vi "JSON File to Cluster.vi"(7 "Cluster (Data Type)":variant, 11 "JSON Document":path) -> (2 "Data":variant)   [LabVIEW 2013]
uses:
  <vilib>/addons/JSON API/JSON Value/JSON Value.lvclass
  <vilib>/addons/JSON API/JSON Value/Set from JSON string.vi
  <vilib>/addons/JSON API/Variant JSON/Get as Variant.vi
  <vilib>/addons/JSON API/Get Polymorphic/JSON GetSet.lvlib
  <vilib>/addons/JSON API/Variant JSON/Variant JSON.lvlib
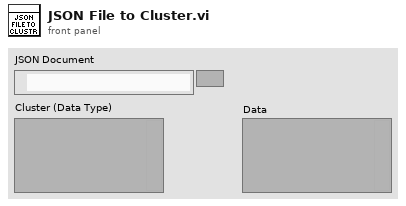
[diagram p1: front panel]
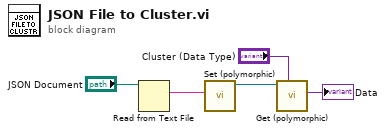
[diagram p0: block diagram]
diagram:
  n1 = Read from Text File(file (use dialog)="JSON Document") -> (text=w4:string)  [unwired: 3 in, 3 out]
  n2 = call-poly <vilib>:"Set (polymorphic).vi"("JSON stream"=w4) -> ("JSON Value out"=w5:refnum<class "JSON Value.lvclass">)  [unwired: 8 in, 2 out]
  n3 = call-poly <vilib>:"Get (polymorphic).vi"("Variant (Data Type)"="Cluster (Data Type)", "JSON Scalar in"=w5) -> ("Variant out"=→"Data":variant)  [unwired: 7 in, 2 out]
